vi "OPC Read Update to Cluster.vi"(7 "Controls[]":refnum<vi>[](array[refnum]), 8 "error in (no error)":errorcluster, 11 "Variant in":variant) -> (0 "error out":errorcluster, 3 "Variant out":variant)   [LabVIEW 2020]
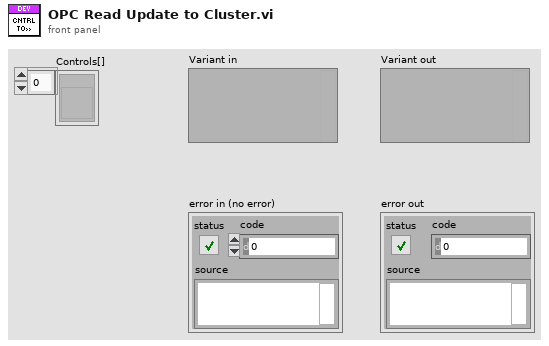
[diagram p1: front panel]
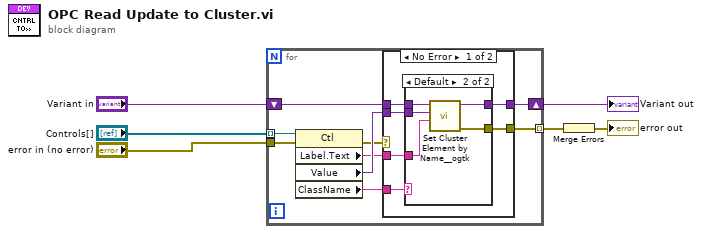
[diagram p0: block diagram]
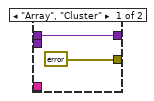
[diagram p2: hidden frame]
diagram:
  n1 = for {
    tunnel: "Controls[]" -> [w10] mode=indexing
    tunnel: "error in (no error)" -> [w9]
    shift-right: [w12] -> w6
    shift-left: "Variant in" -> [w15]
    tunnel: [w11] -> w4 mode=indexing
    n2 = property class="Ctl"(reference=w10, error in=w9) -> (error out=w13:errorcluster, "Label.Text"=w8:string, "Value"=w14:variant, "ClassName"=w7:string)  [unwired: 1 out]
    n3 = case shown="No Error" w13 {
      selector: w13 -> [_ w29]
      tunnel: w15 -> [w21 w30]
      tunnel: w8 -> [w20 _]
      tunnel: w14 -> [w19 _]
      tunnel: [w18 w30] -> w12
      tunnel: [w17 w29] -> w11
      tunnel: w7 -> [w16 _]
      frame No Error {
        n4 = case shown="Default" w16 {
          tunnel: w21 -> [w23 w28]
          tunnel: w20 -> [_ w27]
          tunnel: w19 -> [_ w26]
          tunnel: [w23 w25] -> w18
          tunnel: [errorcluster {"status"=FALSE, "code"=0, "source"=""} ("error out") w24] -> w17
          frame "Array", "Cluster" {
          }
          frame Default {
            n5 = call <userlib>:"Set Cluster Element by Name__ogtk.vi"("Element Name (\"\": New Element Data Name)"=w27, "New Element Value"=w26, "Cluster"=w28) -> ("error out"=w24:errorcluster, "VCluster out"=w25:variant)  [unwired: 6 in, 1 out]
          }
        }
      }
      frame Error {
      }
    }
  }
  "Variant out" <- w6
  n6 = Merge Errors(w4) -> (→"error out":errorcluster)
